vi "MainNR.vi"(10 "JQMHStartup":refnum<class "RQMHStartup.lvclass">, 11 "NewTemplate in":refnum<class "Layout.lvclass">) -> ()   [LabVIEW 2024, in "Layout.lvclass"]
uses:
  Layout.lvclass
  C:/Github/JQMH/JQMHCore/Module/RQMHModule.lvclass
  JQMHCore/JQMHStartup/RQMHStartup.lvclass
  <vilib>/Utility/traverseref.llb/TRef TravTarget.ctl
  Message Queue_class/RQMHMessageQueue.lvclass/RQMHMessageQueue.ctl
  JQMHCore/Module/InitialiseReplyArgs.ctl
  JQMHCore/Module/RQMHModule.lvclass/RQMHModule.ctl
  Do Something ReplyArgs.ctl
  Do Something Args.ctl
  Get SubPanel ReplyArgs.ctl
  Get SubPanel Args.ctl
  JQMHCore/Module/Read ModuleName.vi
  JQMHCore/Module/Read External Start.vi
  Message Queue_class/Delacor_lib_QMH_Enqueue Message (Single).vi
  Message Queue_class/RQMHMessageQueue.lvclass
  JQMHCore/Module/RQMHModule.lvclass
  JQMHCore/Shared/RQMHShared.lvlib
  <vilib>/Utility/traverseref.llb/VI Scripting - Traverse.lvlib
panel:
  out "error out":errorcluster
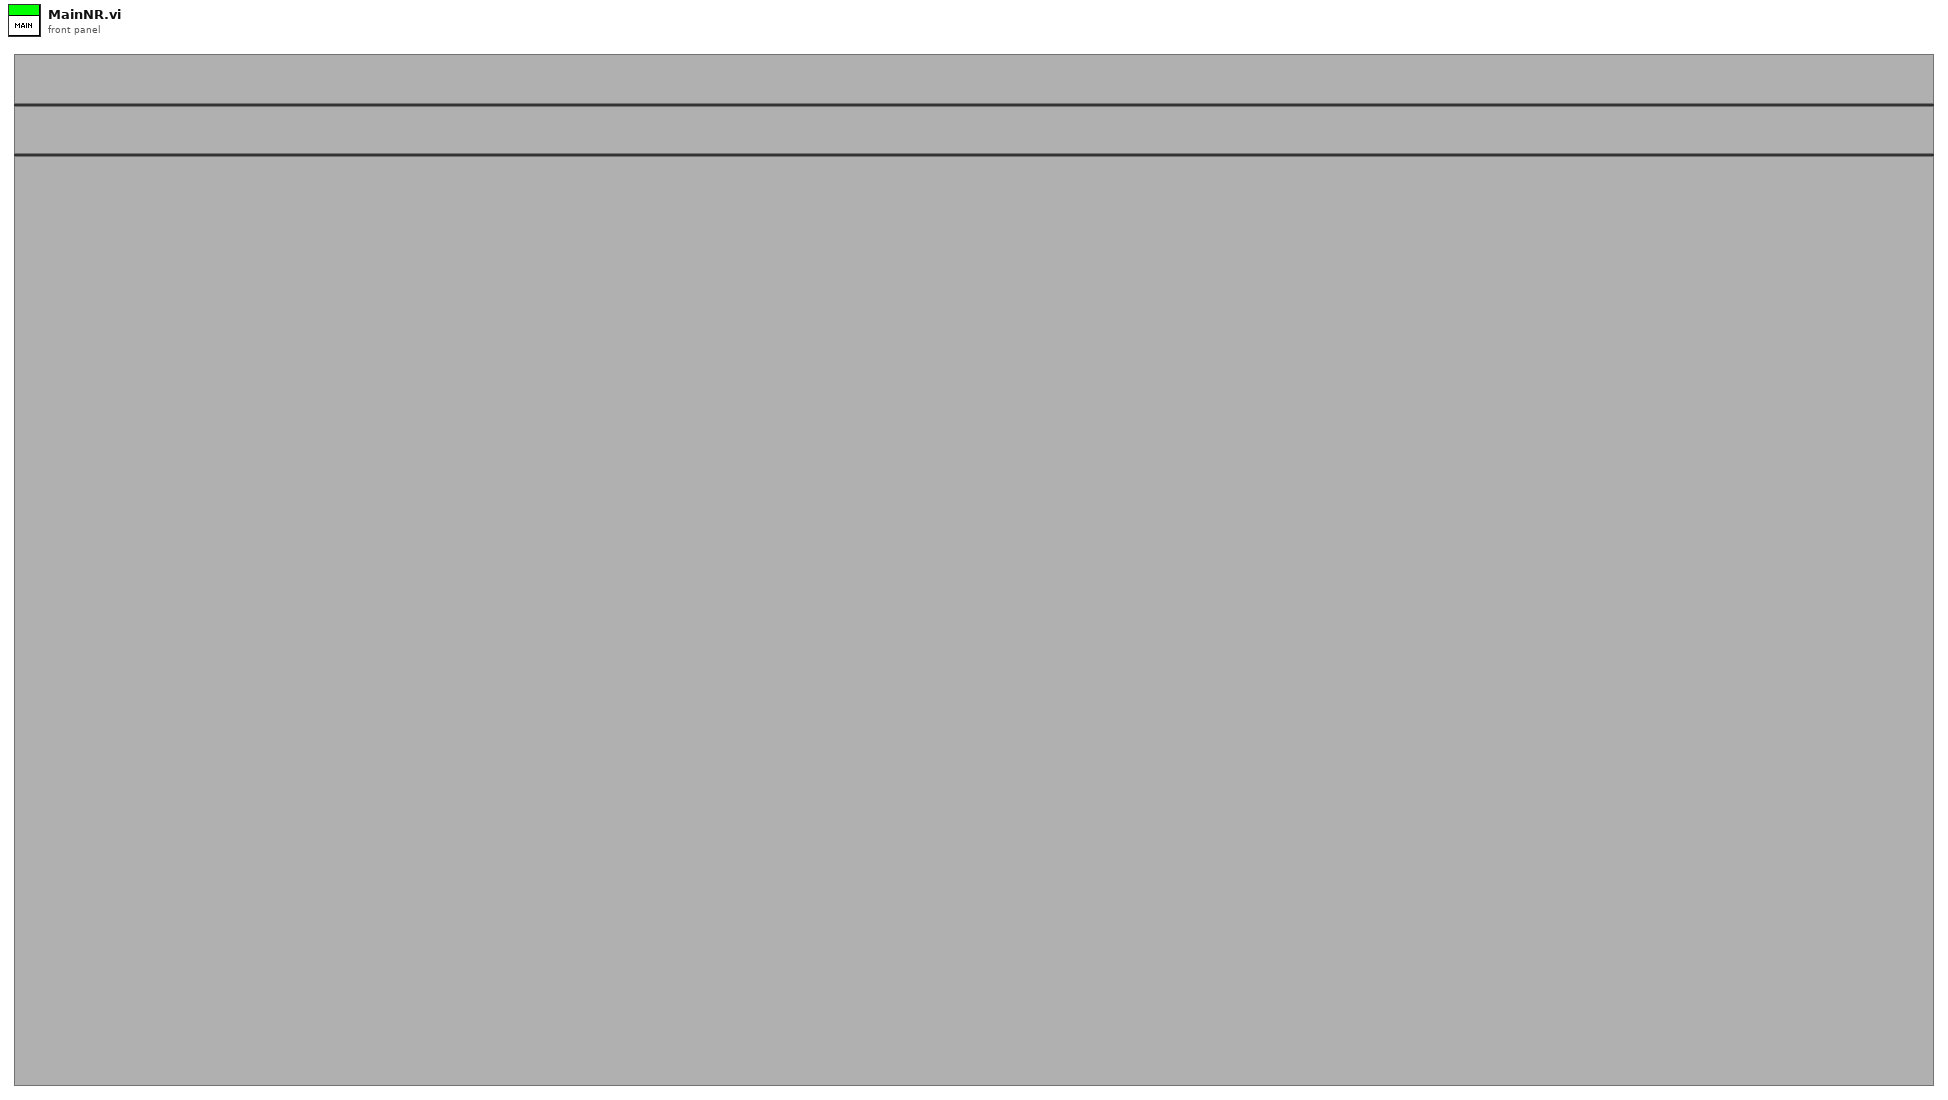
[diagram p1: front panel]
types:
  T1 = typedef "TRef TravTarget.ctl" = enum16{"FP", "BD", "Other"}
  T2 = typedef "Layout.lvclass/Request Events--cluster.ctl" = cluster{"Do Something":refnum<user-event>, "Get SubPanel":refnum<user-event>}
  T3 = cluster{"Stop Module":refnum<user-event>, "Requests":T2}
  T4 = enum32{"Invalid", "Standard", "Closed", "Hidden", "Minimized", "Maximized"}
  T5 = typedef "RQMHModule.lvclass/InitialiseReplyArgs.ctl" = cluster{"Did Init?":bool}
  T6 = typedef "Layout.lvclass/Do Something Args.ctl" = cluster{"Msg":string}
  T7 = typedef "Layout.lvclass/Do Something ReplyArgs.ctl" = cluster{"Value":dbl, "Boolean":bool}
  T8 = typedef "Layout.lvclass/Get SubPanel Args.ctl" = cluster{"Panel Name":string}
  T9 = typedef "Layout.lvclass/Get SubPanel ReplyArgs.ctl" = cluster{"Sub Panel":refnum<vi>}
  T10 = typedef "RQMHModule.lvclass/Reply.ctl" = cluster{"Expects Reply":bool, "Reply":refnum<notifier>}
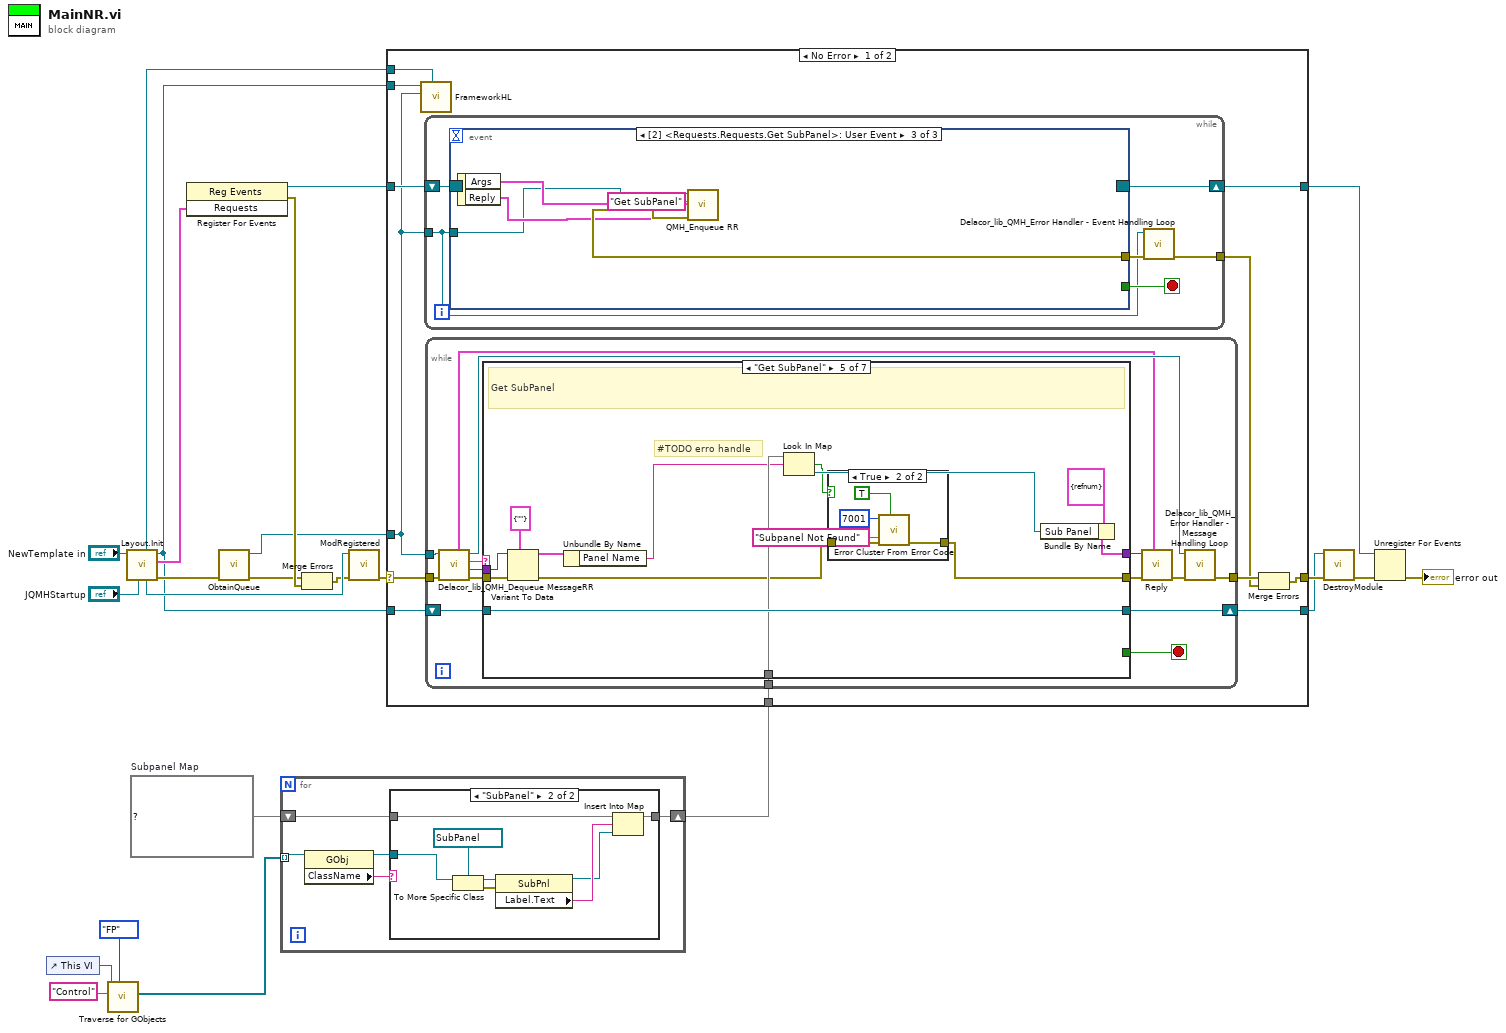
[diagram p0: block diagram]
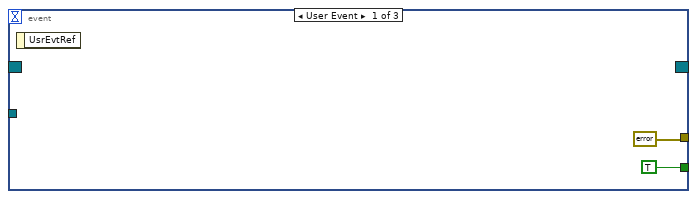
[diagram p3: hidden frame]
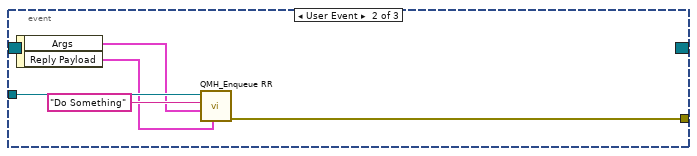
[diagram p4: hidden frame]
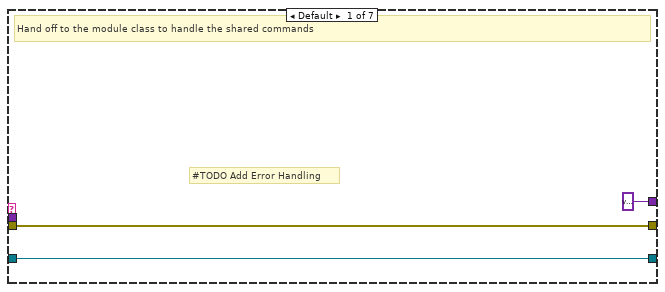
[diagram p5: hidden frame]
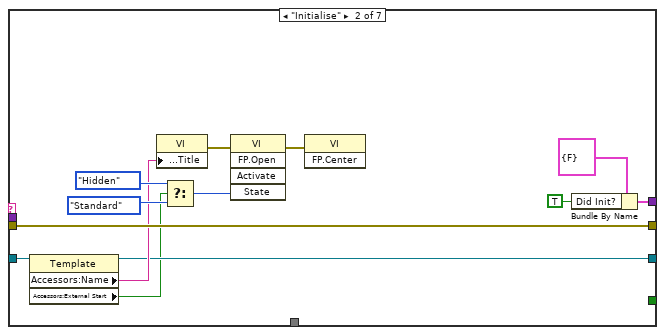
[diagram p6: hidden frame]
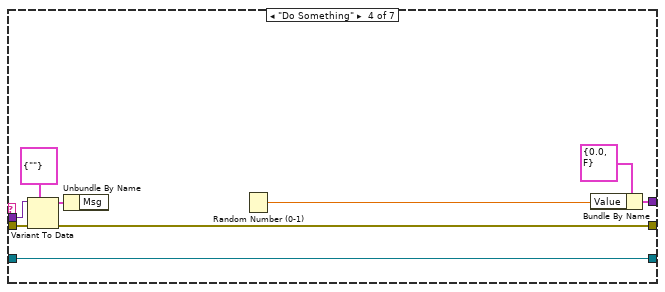
[diagram p8: hidden frame]
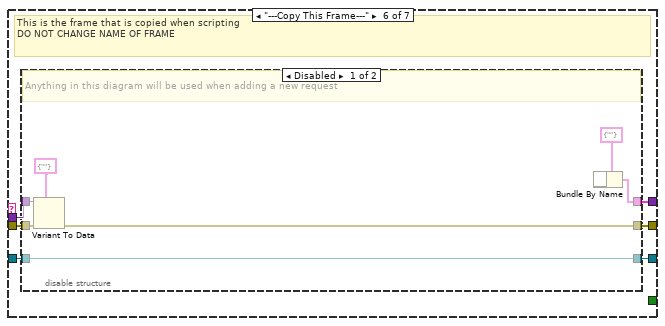
[diagram p10: hidden frame]
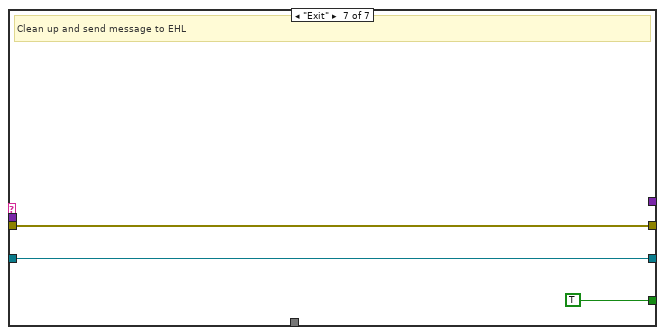
[diagram p12: hidden frame]
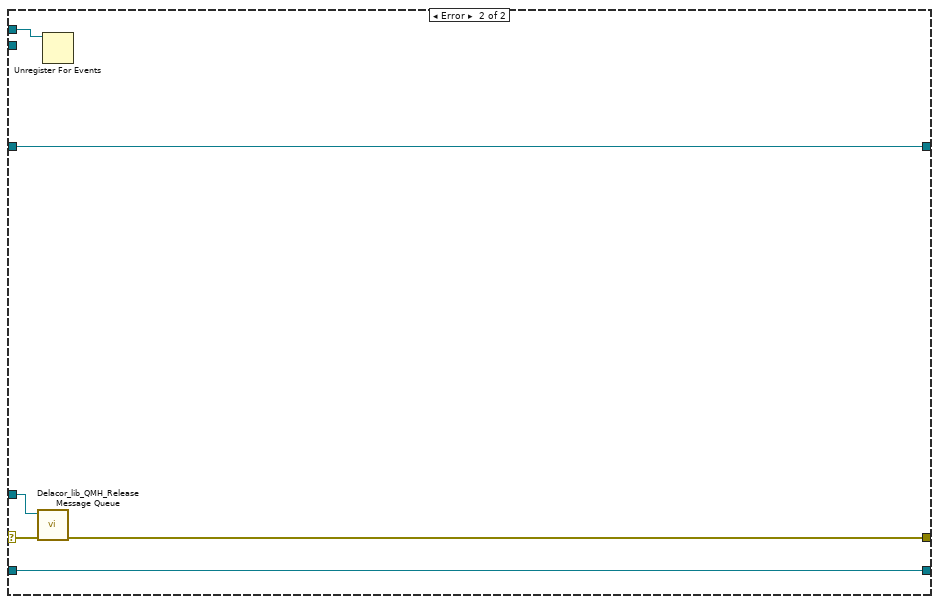
[diagram p13: hidden frame]
diagram:
  w6 = map{string, refnum<vi>} {}  # Subpanel Map
  n1 = control-ref of="This VI"() -> (w1:refnum<vi>)
  n2 = call <vilib>:"Traverse for GObjects.vi"("Traverse Target"=TRef_TravTarget."FP", "Class Name"="Control", "VI Refnum"=w1) -> ("References"=w3:refnum<vi>[])  [unwired: 5 in, 3 out]
  n3 = call "Layout.Init.vi"("JQMHStartup in"="JQMHStartup", "NewTemplate in"="NewTemplate in") -> ("error out"=w17:errorcluster, "Requests"=w8:T3, "NewTemplate out"=w7:refnum<class "Layout.lvclass">, "JQMHStartup out"=w15:refnum<class "RQMHStartup.lvclass">, "StandardRequests"=w11:refnum<event-registration>)  [unwired: 4 in, 1 out]
  n4 = register-events(w8) -> (reference out=w10:refnum<event-registration>, error out=w24:errorcluster)  [unwired: 2 in]
  n5 = call "ObtainQueue.vi"("error in"=w17) -> ("error out"=w16:errorcluster, "Message Queue"=w12:refnum<class "RQMHMessageQueue.lvclass">)  [unwired: 9 in]
  n6 = for {
    tunnel: w3 -> [w29] mode=indexing
    shift-right: [w25] -> w2
    shift-left: w6 -> [w26]
    n7 = property class="GObj"(reference=w29) -> (reference out=w27:refnum<vi>, "ClassName"=w28:string)  [unwired: 1 in, 1 out]
    n8 = case shown="\"SubPanel\"" w28 {
      tunnel: w27 -> [_ w33]
      tunnel: w26 -> [w30 w32]
      tunnel: [w30 w31] -> w25
      frame Default {
      }
      frame "SubPanel" {
        n9 = To More Specific Class(target class=refnum<vi> refnum ("reference out"), reference=w33) -> (specific class reference=w37:refnum<vi>, error out=w36:errorcluster)  [unwired: 1 in]
        n10 = property class="SubPnl"(reference=w37, error in=w36) -> (reference out=w34:refnum<vi>, "Label.Text"=w35:string)  [unwired: 1 out]
        n11 = Insert Into Map(map in=w32, key=w35, value=w34) -> (map out=w31:map{string, refnum<vi>})  [unwired: 2 out]
      }
    }
  }
  n12 = Merge Errors(w16, w24) -> (w13:errorcluster)
  n13 = call "ModRegistered.vi"("error in (no error)"=w13, "JQMHStartup in"=w15) -> ("error out"=w14:errorcluster)  [unwired: 9 in]
  n14 = case "RQMH_MAIN" shown="No Error" w14 {
    selector: w14 -> [w47 w151]
    tunnel: w7 -> [w50 w150]
    tunnel: [w49 w153] -> w23
    tunnel: w10 -> [w48 w153]
    tunnel: w12 -> [w41 w152]
    tunnel: [w46 w150] -> w9
    tunnel: [w43 w149] -> w20
    tunnel: w7 -> [w42 _]
    tunnel: w11 -> [w40 w148]
    tunnel: w2 -> [w39 _]
    frame No Error {
      n15 = call-dynamic "FrameworkHL.vi"("StandardRequests"=w40, "Message Queue"=w41, "JQMHModule in"=w42) -> ()  [unwired: 9 in]
      n16 = while {
        shift-right: [w56] -> w49
        shift-left: w48 -> [w51]
        tunnel: w41 -> [w52]
        tunnel: [w53] -> w44
        stop <- w55 stop-if-true
        n17 = event "RQMH_EVENT_MAIN" shown="[2] <Requests.Requests.Get SubPanel>: User Event" {
          selector: w51 -> [_ _ _]
          dyn-events: [_ _ _] -> w56
          timeout: _ -> [_ _ _]
          tunnel: [TRUE _ _] -> w55
          tunnel: w52 -> [_ w63 w65]
          tunnel: [errorcluster {"status"=FALSE, "code"=0, "source"=""} ("error out") w60 w68] -> w54
          event User Event {
            n18 = event-data() -> ()  [unwired: 1 in, 1 out]
          }
          event User Event {
            n19 = event-data() -> ("Args"=w61:T6, "Reply Payload"=w59:T10)  [unwired: 1 in]
            n20 = call "QMH_Enqueue RR.vi"("Reply"=w59, "Message Data"=w61, "Message"="Do Something", "Message Queue in"=w63) -> ("error out"=w60:errorcluster)  [unwired: 6 in, 1 out]
          }
          event User Event {
            n21 = event-data() -> ("Args"=w66:T8, "Reply"=w67:T10)  [unwired: 1 in]
            n22 = call "QMH_Enqueue RR.vi"("Reply"=w67, "Message Data"=w66, "Message"="Get SubPanel", "Message Queue in"=w65) -> ("error out"=w68:errorcluster)  [unwired: 6 in, 1 out]
          }
        }
        n23 = call-dynamic "Delacor_lib_QMH_Error Handler - Event Handling Loop.vi"("error in"=w54, "Message Queue in"=w52) -> ("dup error in"=w53:errorcluster)  [unwired: 8 in, 1 out]
      }
      n24 = while {
        tunnel: w41 -> [w78]
        tunnel: w47 -> [w77]
        shift-right: [w80] -> w46
        shift-left: w50 -> [w81]
        tunnel: [w79] -> w45
        tunnel: w39 -> [w69]
        stop <- w83 stop-if-true
        n25 = call-dynamic "Delacor_lib_QMH_Dequeue MessageRR.vi"("error in"=w77, "Message Queue in"=w78) -> ("error out"=w76:errorcluster, "Message Data"=w74:variant, "Message"=w75:string, "Message Queue out"=w82:refnum<class "RQMHMessageQueue.lvclass">, "Reply"=w70:T10)  [unwired: 5 in]
        n26 = case "RQMH_MESSAGE_CASES" shown="\"Get SubPanel\"" w75 {
          tunnel: [_ _ _ _ _ _ TRUE] -> w83
          tunnel: w81 -> [w85 w88 w100 w110 w122 w133 w146]
          tunnel: w74 -> [_ _ _ w106 w121 w131 _]
          tunnel: w76 -> [w86 w99 w101 w105 w123 w135 w145]
          tunnel: [w86 w99 w101 w104 w111 w134 w145] -> w73
          tunnel: [w85 w89 w100 w110 w122 w132 w146] -> w80
          tunnel: [variant w98 _ w109 w120 w130 _] -> w71
          tunnel: w69 -> [_ _ _ _ w117 _ _]
          frame Default {
            # "#TODO Add Error Handling"
            # "Hand off to the module class to handle the shared commands"
          }
          frame "Initialise" {
            n27 = property class="Template"(reference=w88) -> (reference out=w89:refnum<class "Layout.lvclass">, "Accessors:Name"=w90:string, "Accessors:External Start"=w87:bool)  [unwired: 1 in, 1 out]
            n28 = property on="Property Node" class="VI"("Front Panel.Title"=w90) -> (error out=w96:errorcluster)  [unwired: 2 in, 1 out]
            n29 = Select(t=T4."Hidden" ("State"), s=w87, f=T4."Standard" ("State")) -> (s? t:f=w92:T4)
            n30 = invoke on="Invoke Node" class="VI" method="FP.Open"(error in=w96, "State"=w92) -> (error out=w95:errorcluster)  [unwired: 3 in, 4 out]
            n31 = invoke on="Invoke Node" class="VI" method="FP.Center"(error in=w95) -> ()  [unwired: 2 in, 3 out]
            n32 = Bundle By Name(cluster=T5 {"Did Init?"=FALSE} ("Args"), "Did Init?"=TRUE) -> (w98:T5)
          }
          frame "---Module Specific---" {
          }
          frame "Do Something" {
            n33 = Variant To Data(error in=w105, type=T6 {"Msg"=""} ("Do Something Args"), Variant=w106) -> (data=w102:T6, error out=w104:errorcluster)
            n34 = Unbundle By Name(w102) -> ()  [unwired: 1 out]
            n35 = Random Number (0-1)() -> (number: 0 to 1=w107:dbl)
            n36 = Bundle By Name(cluster=T7 {"Value"=0.0, "Boolean"=FALSE}, "Value"=w107) -> (w109:T7)
          }
          frame "Get SubPanel" {
            # "#TODO erro handle"
            # "Get SubPanel"
            n37 = Variant To Data(error in=w123, type=T8 {"Panel Name"=""} ("RQMH_MHL_MSG_PL"), Variant=w121) -> (data=w116:T8, error out=w112:errorcluster)
            n38 = Unbundle By Name(w116) -> ("Panel Name"=w115:string)
            n39 = Look In Map(map=w117, key=w115) -> (key not found?=w113:bool, value=w114:refnum<vi>)  [unwired: 1 in]
            n40 = case shown="True" w113 {
              tunnel: w112 -> [w124 w129]
              tunnel: [w124 w128] -> w111
              frame False {
              }
              frame True {
                n41 = call <vilib>:"Error Cluster From Error Code.vi"("show call chain? (False)"=TRUE, "error in (no error)"=w129, "error message (\"\")"="Subpanel Not Found" ("error message (\"\")"), "error code (0)"=7001) -> ("error out"=w128:errorcluster)  [unwired: 5 in]
              }
            }
            n42 = Bundle By Name(cluster=T9 {"Sub Panel"=refnum} ("RQMH_MHL_REPLY_PL"), "Sub Panel"=w114) -> (w120:T9)
          }
          frame "---Copy This Frame---" {
            # "This is the frame that is copied when scripting\nDO NOT CHANGE NAME OF FRAME"
            n43 = disable-structure shown="Disabled" {
              disable-tunnel: w135 -> [w139 w144]
              disable-tunnel: [w140 w144] -> w134
              disable-tunnel: w133 -> [w142 w143]
              disable-tunnel: [w142 w143] -> w132
              disable-tunnel: w131 -> [w141 _]
              disable-tunnel: [w137 _] -> w130
              frame Disabled {
                # "Anything in this diagram will be used when adding a new request"
                n44 = Variant To Data(error in=w139, type=cluster{string} {""} ("RQMH_MHL_MSG_PL"), Variant=w141) -> (error out=w140:errorcluster)  [unwired: 1 out]
                n45 = Bundle By Name(cluster=cluster{string} {""} ("RQMH_MHL_REPLY_PL")) -> (w137:cluster{string})  [unwired: 1 in]
              }
              frame Enabled {
              }
            }
          }
          frame "Exit" {
            # "Clean up and send message to EHL"
          }
        }
        n46 = call "Reply.vi"("Reply"=w70, "error in (no error)"=w73, "ReplyPayload"=w71) -> ("error out"=w72:errorcluster)  [unwired: 8 in]
        n47 = call-dynamic "Delacor_lib_QMH_Error Handler - Message Handling Loop.vi"("error in"=w72, "Message Queue in"=w82) -> ("dup error in"=w79:errorcluster)  [unwired: 8 in, 1 out]
      }
      n48 = Merge Errors(w45, w44) -> (w43:errorcluster)
    }
    frame Error {
      n49 = call-dynamic "Delacor_lib_QMH_Release Message Queue.vi"("error in"=w151, "Message Queue"=w152) -> ("error out"=w149:errorcluster)  [unwired: 9 in]
      n50 = Unregister For Events(event registration refnum=w148) -> ()  [unwired: 1 in, 1 out]
    }
  }
  n51 = call "DestroyModule.vi"("error in (no error)"=w20, "JQMHModule in"=w9) -> ("error out"=w22:errorcluster)  [unwired: 9 in]
  n52 = Unregister For Events(event registration refnum=w23, error in=w22) -> (error out=→"error out":errorcluster)
